vi "Pool motor status.vi"(0 "Update Motors Notifier":refnum<notifier>, 1 "Right motor Clustered SDO":T1, 2 "Left motor Clustered SDO":T1, 7 "Error Queue":refnum<queue>) -> (21 "Left Motor Status":T3, 22 "Left Motor Statusword":T4, 23 "Right Motor Status":T3, 24 "Right Motor Statusword":T4, 27 "Exit?":bool)   [LabVIEW 2016]
uses:
  RT/Statusword.ctl
  RT/Clustered SDO.ctl
  RT/Get Motor Status.vi
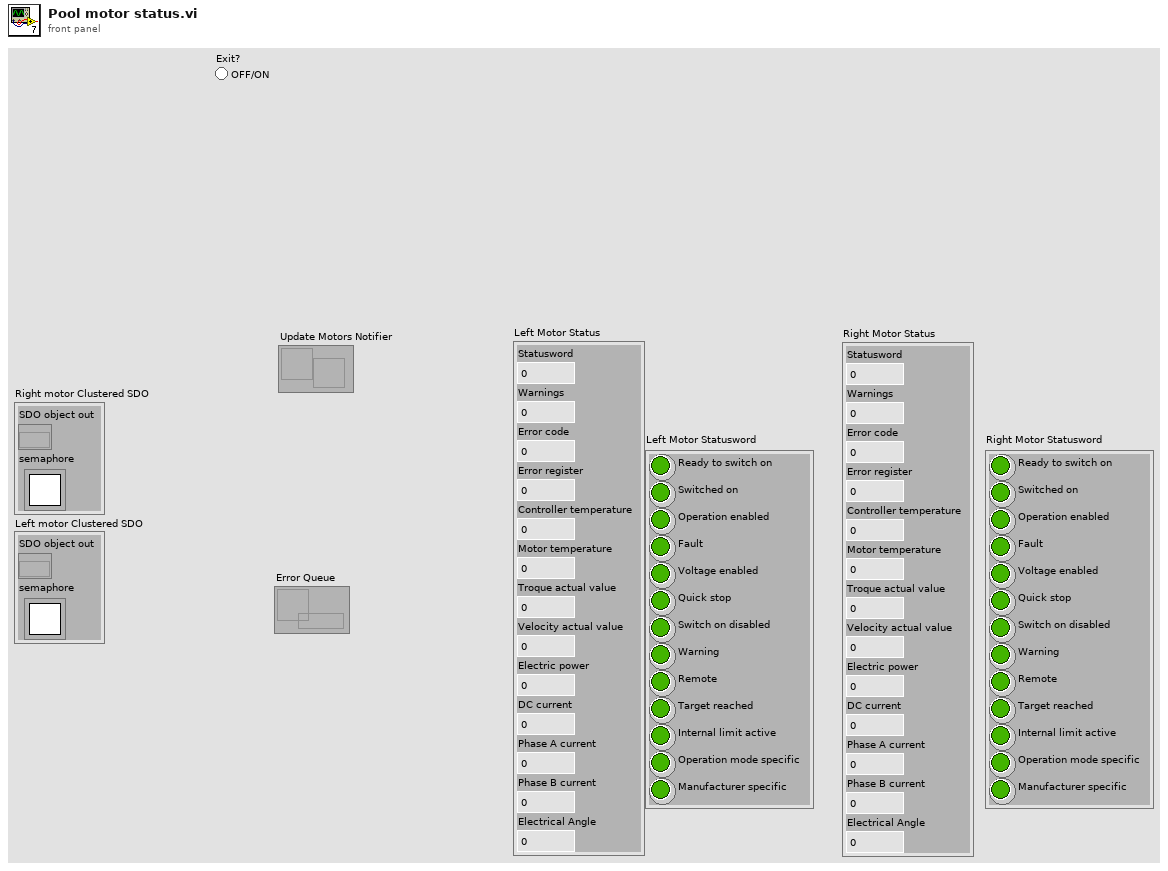
[diagram p1: front panel]
types:
  T1 = typedef "Clustered SDO.ctl" = cluster{"SDO object out":refnum<k20>, "semaphore":T2}
  T2 = typedef "Semaphore RefNum" = refnum<k1>
  T3 = cluster{"Statusword":u16, "Warnings":u16, "Error code":u16, "Error register":u8, "Controller temperature":u8, "Motor temperature":u8, "Troque actual value":i16, "Velocity actual value":i32, "Electric power":u32, "DC current":u32, "Phase A current":u16, "Phase B current":u16, "Electrical Angle":u16}
  T4 = typedef "Statusword.ctl" = cluster{"Ready to switch on":bool, "Switched on":bool, "Operation enabled":bool, "Fault":bool, "Voltage enabled":bool, "Quick stop":bool, "Switch on disabled":bool, "Warning":bool, "Remote":bool, "Target reached":bool, "Internal limit active":bool, "Operation mode specific":bool, "Manufacturer specific":bool}
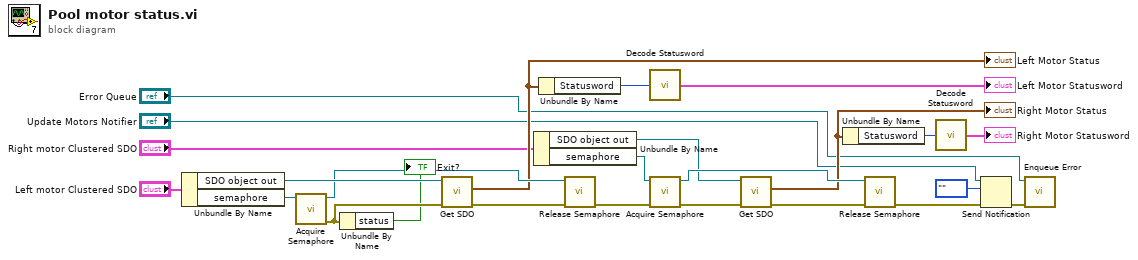
[diagram p0: block diagram]
diagram:
  n1 = Unbundle By Name("Left motor Clustered SDO") -> ("SDO object out"=w23:refnum<k20>, "semaphore"=w24:T2)
  n2 = call <vilib>:"Acquire Semaphore.vi"("semaphore"=w24) -> ("error out"=w6:errorcluster, "semaphore out"=w21:T2)  [unwired: 4 in, 1 out]
  n3 = Unbundle By Name(w6) -> ("status"=→"Exit?":bool)
  n4 = call-poly "Get SDO.vi"("error in (no error)"=w6, "SDO object in"=w23) -> ("error out"=w22:errorcluster, "Motor Status"=w20:T3)  [unwired: 7 in, 1 out]
  "Left Motor Status" <- w20
  n5 = Unbundle By Name("Right motor Clustered SDO") -> ("SDO object out"=w14:refnum<k20>, "semaphore"=w13:T2)
  n6 = Unbundle By Name(w20) -> ("Statusword"=w19:u16)
  n7 = call <vilib>:"Release Semaphore.vi"("error in (no error)"=w22, "semaphore"=w21) -> ("error out"=w11:errorcluster)  [unwired: 4 in, 1 out]
  n8 = call "Decode Statusword.vi"("Data"=w19) -> ("Status"=→"Left Motor Statusword":T4)
  n9 = call <vilib>:"Acquire Semaphore.vi"("error in (no error)"=w11, "semaphore"=w13) -> ("error out"=w12:errorcluster, "semaphore out"=w16:T2)  [unwired: 3 in, 1 out]
  n10 = call-poly "Get SDO.vi"("error in (no error)"=w12, "SDO object in"=w14) -> ("error out"=w15:errorcluster, "Motor Status"=w8:T3)  [unwired: 7 in, 1 out]
  "Right Motor Status" <- w8
  n11 = Unbundle By Name(w8) -> ("Statusword"=w17:u16)
  n12 = call <vilib>:"Release Semaphore.vi"("error in (no error)"=w15, "semaphore"=w16) -> ("error out"=w10:errorcluster)  [unwired: 4 in, 1 out]
  n13 = call "Decode Statusword.vi"("Data"=w17) -> ("Status"=→"Right Motor Statusword":T4)
  n14 = Send Notification(notification=enum16{""}."", notifier="Update Motors Notifier", error in (no error)=w10) -> (error out=w7:errorcluster)  [unwired: 1 out]
  n15 = call "Enqueue Error.vi"("error in"=w7, "Error Queue"="Error Queue") -> ()  [unwired: 10 in]
